vi "Open Connection.vi"(8 "error in (no error)":errorcluster) -> (0 "error out":errorcluster, 2 "connection reference":T1)   [LabVIEW 2016, in "Data Saving.lvlib" / "SQL Saver.lvclass"]
uses:
  SQL Saver.lvclass
  <vilib>/addons/database/Connection.llb/Conn ObjectReference.ctl
  <vilib>/addons/database/Connection.llb/DB Tools Open Connec (String).vi
  <vilib>/addons/database/NI_Database_API.lvlib
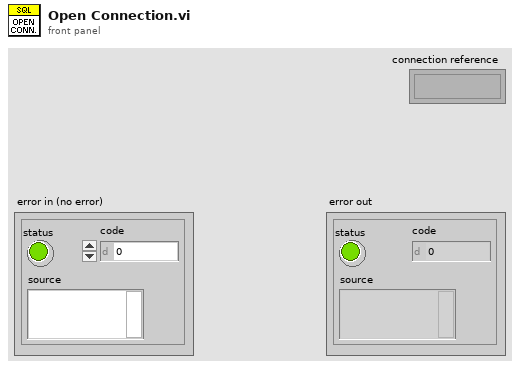
[diagram p1: front panel]
types:
  T1 = typedef "NI_Database_API.lvlib/Conn ObjectReference.ctl" = refnum<k1>
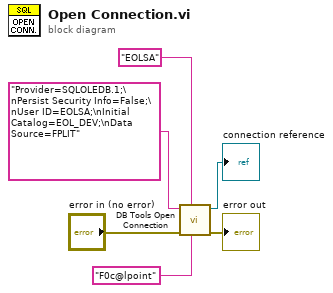
[diagram p0: block diagram]
diagram:
  n1 = call-poly <vilib>:"DB Tools Open Connection.vi"("password"="F0c@lpoint", "userID"="EOLSA", "error in (no error)"="error in (no error)", "connection information"="Provider=SQLOLEDB.1;\nPersist Security Info=False;\nUser ID=EOLSA;\nInitial Catalog=EOL_DEV;\nData Source=FPLIT" ("ConnectionString")) -> ("error out"=→"error out":errorcluster, "connection reference"=→"connection reference":T1)  [unwired: 4 in]
